vi "cs_RS232TMC_write.vi"(7 "ParseCMD?":bool, 8 "error in (no error)":errorcluster, 10 "command":string, 11 "Variant In":variant) -> (0 "error out":errorcluster, 3 "variant Out":variant)   [LabVIEW 2024]
uses:
  <vilib>/Instr/_visa.llb/VISA Flush IO Buffer Mask.ctl
panel:
  out "Error":bool
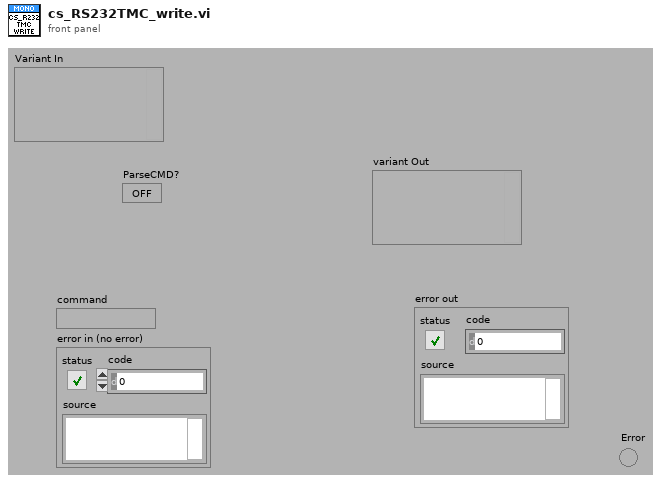
[diagram p1: front panel]
types:
  T1 = typedef "VISA Flush IO Buffer Mask.ctl" = u16
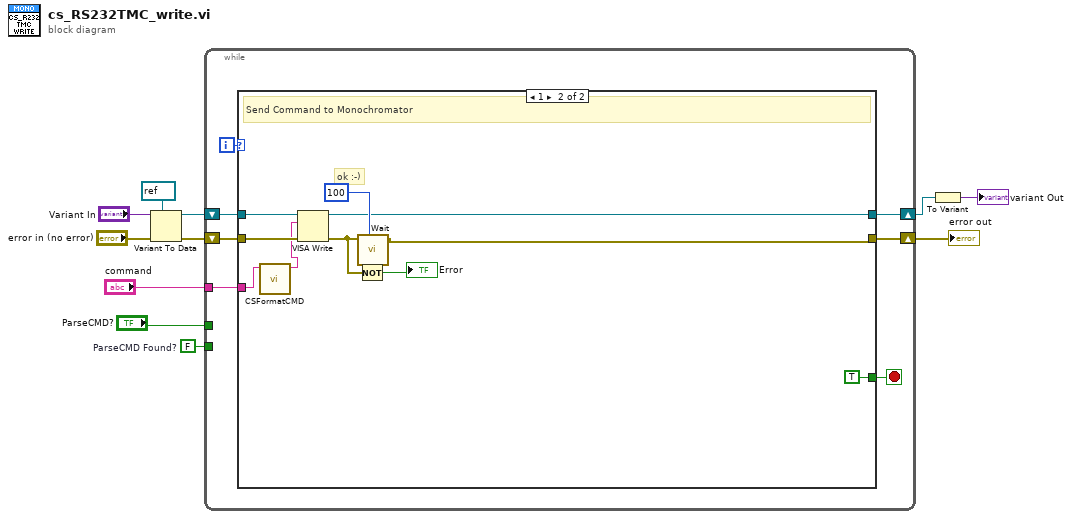
[diagram p0: block diagram]
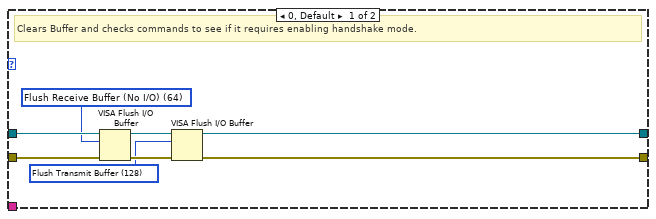
[diagram p2: hidden frame]
diagram:
  w1 = FALSE  # ParseCMD Found?
  n1 = Variant To Data(error in="error in (no error)", type=refnum<visa-resource-name> refnum ("VISA resource name"), Variant="Variant In") -> (data=w7:refnum<visa-resource-name>, error out=w5:errorcluster)
  n2 = while {
    tunnel: "command" -> [w17]
    shift-right: [w16] -> w3
    shift-left: w7 -> [w12]
    shift-right: [w14] -> w10
    shift-left: w5 -> [w15]
    tunnel: "ParseCMD?" -> [_]
    tunnel: w1 -> [_]
    i -> [w18]
    stop <- w13 stop-if-true
    n3 = case shown="1" w18 {
      tunnel: w17 -> [_ w29]
      tunnel: w12 -> [w25 w33]
      tunnel: [w24 w30] -> w16
      tunnel: w15 -> [w26 w34]
      tunnel: [w23 w31] -> w14
      tunnel: [_ TRUE] -> w13
      frame 0, Default {
        w19 = T1 128 items=["Flush Receive Buffer"=16, "Write Transmit Buffer to Device"=32, "Flush Receive Buffer (No I/O)"=64, "Flush Transmit Buffer"=128] ("Mask")
        w22 = T1 64 items=["Flush Receive Buffer"=16, "Write Transmit Buffer to Device"=32, "Flush Receive Buffer (No I/O)"=64, "Flush Transmit Buffer"=128] ("Mask")
        # "Clears Buffer and checks commands to see if it requires enabling handshake mode."
        n4 = VISA Flush I/O Buffer(VISA resource name=w25, mask (16)=w22, error in (no error)=w26) -> (VISA resource name out=w20:refnum<visa-resource-name>, error out=w21:errorcluster)
        n5 = VISA Flush I/O Buffer(VISA resource name=w20, mask (16)=w19, error in (no error)=w21) -> (VISA resource name out=w24:refnum<visa-resource-name>, error out=w23:errorcluster)
      }
      frame 1 {
        # "ok :-)"
        # "Send Command to Monochromator"
        n6 = call "CSFormatCMD.vi"("command in"=w29) -> ("Formated command string"=w28:string)  [unwired: 10 in]
        n7 = VISA Write(VISA resource name=w33, write buffer=w28, error in (no error)=w34) -> (VISA resource name out=w30:refnum<visa-resource-name>, error out=w32:errorcluster)  [unwired: 1 out]
        n8 = Not(x=w32) -> (.not. x?=→"Error":bool)
        n9 = call "Wait.vi"("milliseconds to wait"=u32 100, "Error In"=w32) -> ("Error Out"=w31:errorcluster)  [unwired: 9 in]
      }
    }
  }
  "error out" <- w10
  n10 = To Variant(anything=w3) -> (Variant=→"variant Out":variant)
